vi "Add Sections and Channels.vi"(8 "Error In":errorcluster, 10 "Mux Data Array":T2[](array[typedef]), 11 "Custom Device Ref in":T1 format="%.0x") -> (0 "Error Out":errorcluster, 3 "Custom Device Ref out":T1=18446744073709551615 format="%.0x")   [LabVIEW 2013, in "MUX Custom Device.lvlib"]
uses:
  MUX Custom Device.lvlib
  <vilib>/NI Veristand/Custom Device API/Custom Device Item Ref.ctl
  Mux Data.ctl
  Relay Channel Data.ctl
  Relay Data.ctl
  Switch.ctl
  MUX Global.vi
  <vilib>/NI Veristand/Custom Device API/Custom Device API.lvlib
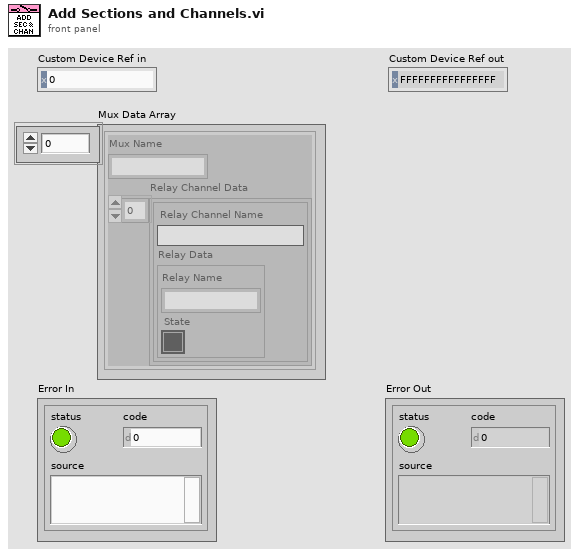
[diagram p1: front panel]
types:
  T1 = typedef "Custom Device API.lvlib/Custom Device Item Ref.ctl" = u64
  T2 = typedef "MUX Custom Device.lvlib/Mux Data.ctl" = cluster{"Mux Name":string, "Relay Channel Data":T3[]}
  T3 = typedef "MUX Custom Device.lvlib/Relay Channel Data.ctl" = cluster{"Relay Channel Name":string, "Relay Data":T4}
  T4 = typedef "MUX Custom Device.lvlib/Relay Data.ctl" = cluster{"Relay Name":string, "State":T5}
  T5 = typedef "MUX Custom Device.lvlib/Switch.ctl" = bool
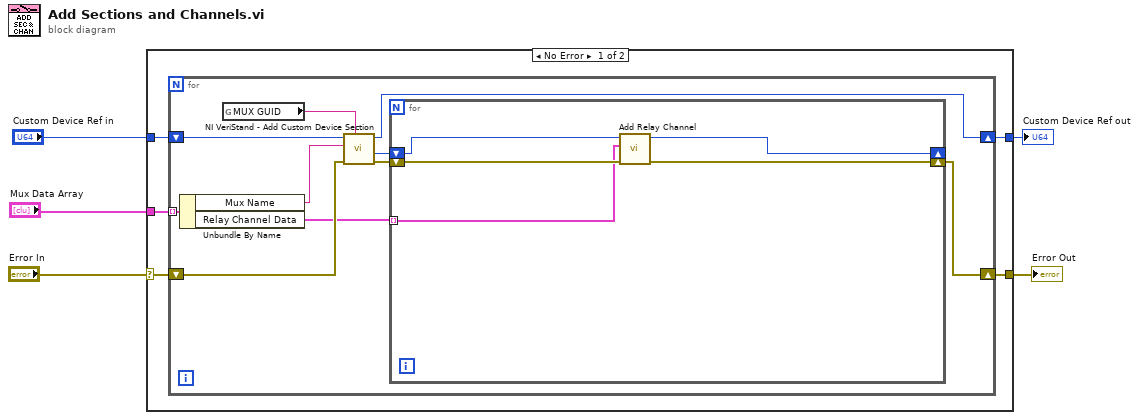
[diagram p0: block diagram]
diagram:
  n1 = case shown="No Error" "Error In" {
    selector: "Error In" -> [w9 w27]
    tunnel: "Custom Device Ref in" -> [w10 w26]
    tunnel: "Mux Data Array" -> [w8 _]
    tunnel: [w7 w27] -> w2
    tunnel: [w6 w26] -> w1
    frame No Error {
      n2 = for {
        tunnel: w8 -> [w18] mode=indexing
        shift-right: [w11] -> w7
        shift-left: w9 -> [w19]
        shift-right: [w13] -> w6
        shift-left: w10 -> [w20]
        n3 = Unbundle By Name(w18) -> ("Mux Name"=w17:string, "Relay Channel Data"=w14:T3[])
        n4 = global read "MUX Global.vi" "MUX GUID"() -> (w12:string)
        n5 = call <vilib>:"NI VeriStand - Add Custom Device Section.vi"("GUID (Default Section)"=w12, "error in (no error)"=w19, "Section Name"=w17, "Parent Ref in"=w20) -> ("error out"=w16:errorcluster, "Section Ptr"=w15:T1, "Parent Ref out"=w13:T1)  [unwired: 4 in, 1 out]
        n6 = for {
          shift-right: [w21] -> w11
          shift-left: w16 -> [w25]
          tunnel: w14 -> [w23] mode=indexing
          shift-right: [w22] -> _
          shift-left: w15 -> [w24]
          n7 = call "Add Relay Channel.vi"("error in (no error)"=w25, "Relay Channel Data"=w23, "MUX Section Ref in"=w24) -> ("error out"=w21:errorcluster, "MUX Section Ref out"=w22:T1)  [unwired: 7 in]
        }
      }
    }
    frame Error {
    }
  }
  "Error Out" <- w2
  "Custom Device Ref out" <- w1
